vi "principal.vi"() -> ()   [LabVIEW 2018]
uses:
  Global 1.vi
panel:
  out "ledstop":bool
  in  "stop":bool
  out "vert":bool
  out "rouge":bool
  out "Trésor":picture
  out "Maximum":dbl
  out "Nb tentatives":dbl
  in  "Ouvrir Button":bool
  in  "3":i8(knob) min=0 max=9 step=1 scale=0.0..10.0
  in  "2":i8(knob) min=0 max=9 step=1 scale=0.0..10.0
  in  "1":i8(knob) min=0 max=9 step=1 scale=0.0..10.0
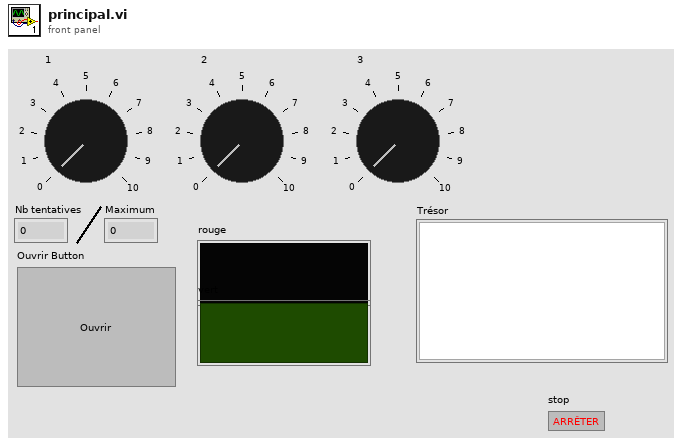
[diagram p1: front panel]
types:
  T1 = enum8{"Enabled", "Disabled", "Disabled and Grayed Out"}
  T2 = typedef "imagedata.ctl" = cluster{"image type":i32, "image depth":i32, "image":u8[], "mask":u8[], "colors":u32[], "Rectangle":cluster{"left":i16, "top":i16, "right":i16, "bottom":i16}}
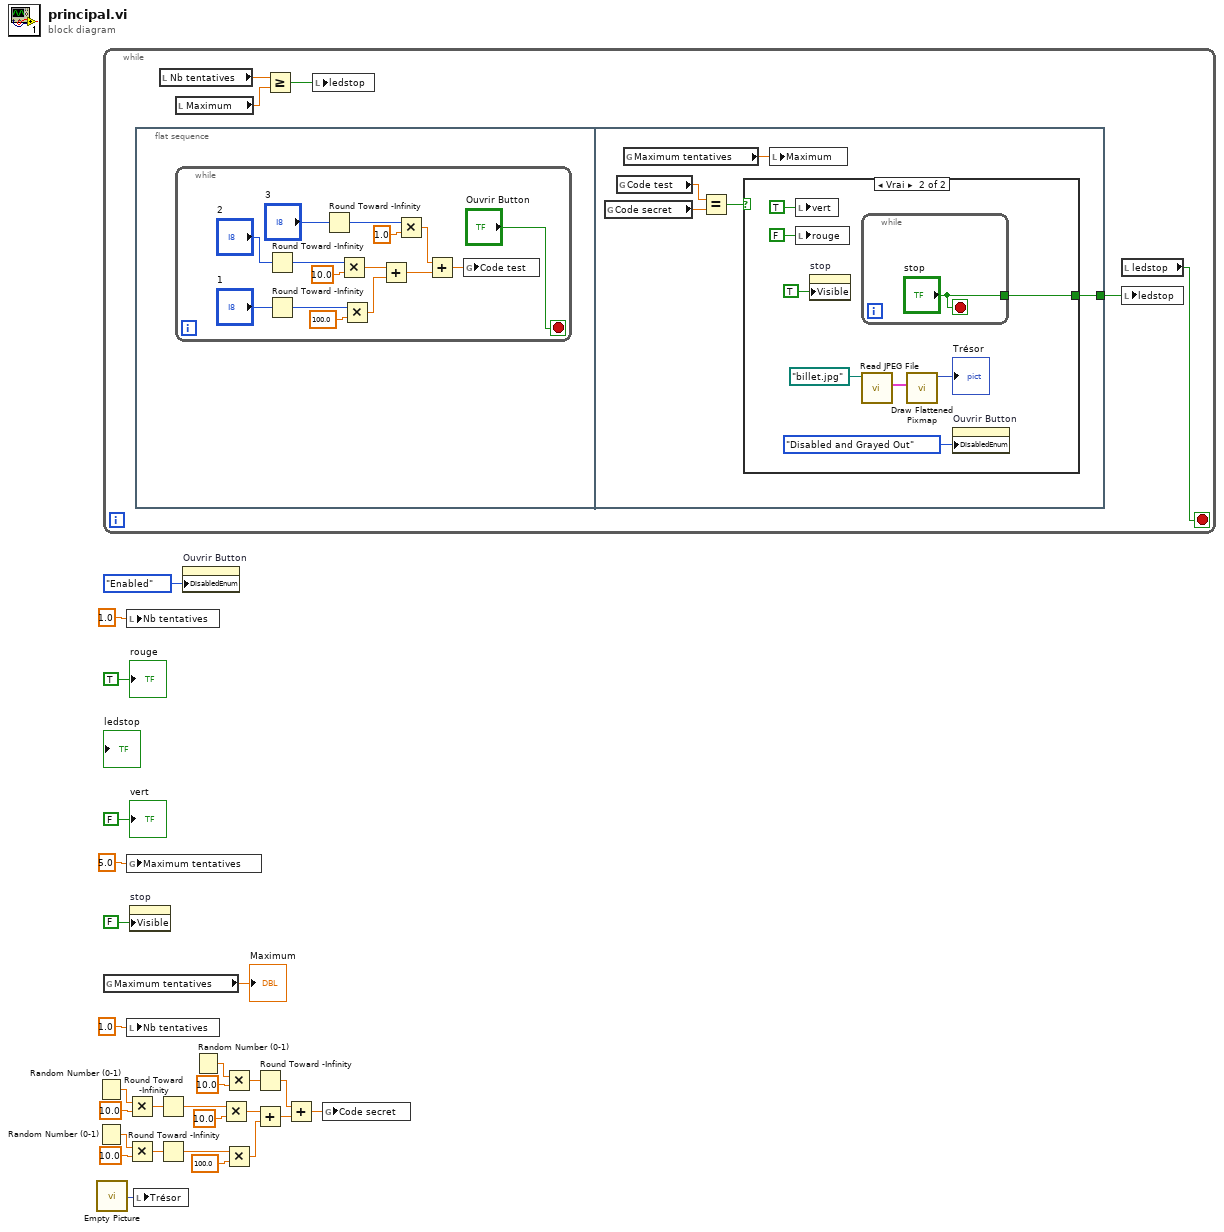
[diagram p0: block diagram]
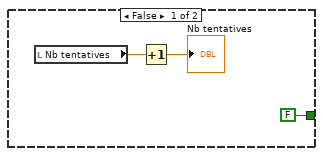
[diagram p2: hidden frame]
diagram:
  n1 = Random Number (0-1)() -> (number: 0 to 1=w24:dbl)
  n2 = Random Number (0-1)() -> (number: 0 to 1=w22:dbl)
  n3 = call "Empty Picture"() -> ("empty picture"=w27:picture)
  n4 = while {
    stop <- w30 stop-if-true
    n5 = flat-sequence {
      tunnel: [w48] -> w28
      frame #0 {
        n6 = while {
          stop <- "Ouvrir Button" stop-if-true
          n7 = Round Toward -Infinity(1:"2") -> (0:w47:i8)
          n8 = Round Toward -Infinity(1:"1") -> (0:w46:i8)
          n9 = Round Toward -Infinity(1:"3") -> (0:w40:i8)
          n10 = Multiply(x=w47, y=10.0) -> (x*y=w45:dbl)
          n11 = Multiply(x=w46, y=100.0) -> (x*y=w44:dbl)
          n12 = Add(x=w45, y=w44) -> (x+y=w37:dbl)
          n13 = Multiply(x=w40, y=1.0) -> (x*y=w35:dbl)
          n14 = Add(x=w35, y=w37) -> (x+y=w36:dbl)
          n15 = global write "Global 1.vi" "Code test"(w36) -> ()
        }
      }
      frame #1 {
        n16 = global read "Global 1.vi" "Code secret"() -> (w50:dbl)
        n17 = global read "Global 1.vi" "Code test"() -> (w51:dbl)
        n18 = global read "Global 1.vi" "Maximum tentatives"() -> (w49:dbl)
        n19 = Equal?(x=w51, y=w50) -> (x = y?=w52:bool)
        n20 = case shown="Vrai" w52 {
          tunnel: [FALSE ("stop") w56] -> w48
          frame False {
            n21 = local read "Nb tentatives"() -> (w55:dbl)
            n22 = Increment(x=w55) -> (x+1=→"Nb tentatives":dbl)
          }
          frame True {
            n23 = local write "vert"(TRUE ("vert")) -> ()
            n24 = local write "rouge"(FALSE ("rouge")) -> ()
            n25 = property on="stop" class="Bool"("Visible"=TRUE) -> ()  [unwired: 2 in, 2 out]
            n26 = while {
              tunnel: ["stop"] -> w56
              stop <- "stop" stop-if-true
            }
            n27 = call <vilib>:"Read JPEG File.vi"("path to JPEG file"=path "billet.jpg") -> ("image data"=w62:T2)  [unwired: 8 in, 2 out]
            n28 = call <vilib>:"Draw Flattened Pixmap.vi"("image data"=w62) -> ("new picture"=→"Trésor":picture)  [unwired: 8 in]
            n29 = property on="Ouvrir Button" class="Bool"("DisabledEnum"=T1."Disabled and Grayed Out" ("Désactivé")) -> ()  [unwired: 2 in, 2 out]
          }
        }
        n30 = local write "Maximum"(w49) -> ()
      }
    }
    n31 = local read "Nb tentatives"() -> (w32:dbl)
    n32 = local read "Maximum"() -> (w31:dbl)
    n33 = Greater Or Equal?(x=w32, y=w31) -> (x >= y?=w29:bool)
    n34 = local write "ledstop"(w29) -> ()
    n35 = local read "ledstop"() -> (w30:bool)
    n36 = local write "ledstop"(w28) -> ()
  }
  n37 = global read "Global 1.vi" "Maximum tentatives"() -> (→"Maximum":dbl)
  n38 = local write "Nb tentatives"(1.0 ("Nb tentatives")) -> ()
  n39 = global write "Global 1.vi" "Maximum tentatives"(5.0 ("Maximum tentatives")) -> ()
  n40 = local write "Nb tentatives"(1.0 ("Nb tentatives")) -> ()
  n41 = Multiply(x=w24, y=10.0) -> (x*y=w23:dbl)
  n42 = Multiply(x=w22, y=10.0) -> (x*y=w21:dbl)
  n43 = property on="stop" class="Bool"("Visible"=FALSE) -> ()  [unwired: 2 in, 2 out]
  n44 = local write "Trésor"(w27) -> ()
  n45 = Round Toward -Infinity(1:w23) -> (0:w20:dbl)
  n46 = Round Toward -Infinity(1:w21) -> (0:w19:dbl)
  n47 = property on="Ouvrir Button" class="Bool"("DisabledEnum"=T1."Enabled" ("Désactivé")) -> ()  [unwired: 2 in, 2 out]
  n48 = Random Number (0-1)() -> (number: 0 to 1=w25:dbl)
  n49 = Multiply(x=w20, y=10.0) -> (x*y=w18:dbl)
  n50 = Multiply(x=w25, y=10.0) -> (x*y=w16:dbl)
  n51 = Multiply(x=w19, y=100.0) -> (x*y=w17:dbl)
  n52 = Round Toward -Infinity(1:w16) -> (0:w14:dbl)
  n53 = Add(x=w18, y=w17) -> (x+y=w15:dbl)
  n54 = Add(x=w14, y=w15) -> (x+y=w13:dbl)
  n55 = global write "Global 1.vi" "Code secret"(w13) -> ()
  "rouge" <- TRUE ("rouge")
  "vert" <- FALSE ("vert")
